vi "checktimeout.vi"(7 "input error":errorcluster) -> (1 "output error":errorcluster, 3 "timeout?":bool)   [LabVIEW 2016]
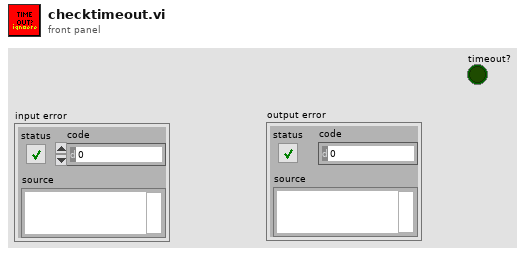
[diagram p1: front panel]
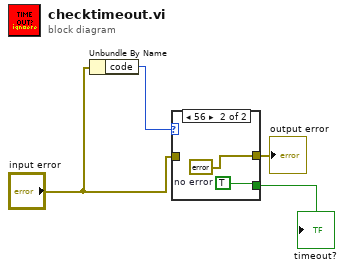
[diagram p0: block diagram]
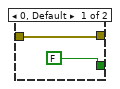
[diagram p2: hidden frame]
diagram:
  n1 = Unbundle By Name("input error") -> ("code"=w4:i32)
  n2 = case shown="56" w4 {
    tunnel: "input error" -> [w6 _]
    tunnel: [w6 w8] -> w2
    tunnel: [FALSE TRUE] -> w1
    frame 0, Default {
    }
    frame 56 {
      w8 = errorcluster {"status"=FALSE, "code"=0, "source"=""}  # no error
    }
  }
  "output error" <- w2
  "timeout?" <- w1
